vi "dswap - Vector Swap (DBL).vi"(5 "yInc":i32=1, 7 "xInc":i32=1, 10 "y":dbl[](array[numeric]), 11 "x":dbl[](array[numeric])) -> (0 "error":i32, 2 "dswap y":dbl[](array[numeric]), 3 "dswap x":dbl[](array[numeric]))   [LabVIEW 2020, in "NI_AALBLAS.lvlib"]
doc: "Swaps elements between two vectors."
uses:
  NI_AALBLAS.lvlib
  Fucntion.ctl
panel:
  # "dswap x=y\ndswap y=x"
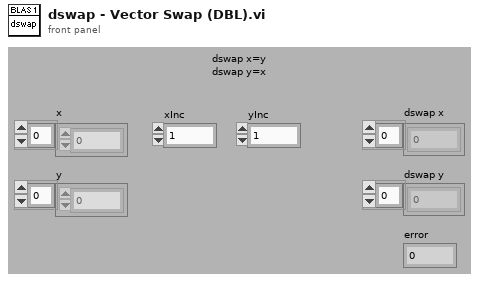
[diagram p1: front panel]
types:
  T1 = typedef "NI_AALBLAS.lvlib/Fucntion.ctl" = u16
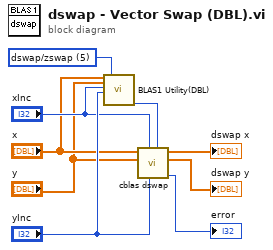
[diagram p0: block diagram]
diagram:
  w1 = T1 5 items=["ddot/zdotu/zdotc", "daxpy/zaxpy", "dnrm2/dznrm2", "dasum/dzasum", "dcopy/zcopy", "dswap/zswap", "drotm", "drot/zdrot", "idamax/izamax", "idamin/izamin", "dgemv/zgemv", "dsymv/zhemv", "dtrmv/ztrmv", "dsyr/zher", "dsyr2/zher2", "dger/zgeru/zgerc", "dtrsv/ztrsv", "dgemm/zgemm", "dsymm/zsymm/zhemm", "dtrmm/ztrmm", "dsyrk/zsyrk/zherk", "dsyr2k/zsyr2k/zher2k", "dtrsm/ztrsm"] ("function")
  n1 = call "BLAS1 Utility(DBL).vi"("x"="x", "y"="y", "xInc"="xInc", "yInc"="yInc", "function"=w1) -> ("n"=w2:i32)  [unwired: 14 in]
  n2 = call "cblas dswap.vi"("n"=w2, "incy"="yInc", "incx"="xInc", "y"="y", "x"="x") -> ("error"=→"error":i32, "dswap y"=→"dswap y":dbl[], "dswap x"=→"dswap x":dbl[])  [unwired: 4 out]
